vi "按日期零件型号保存图片.vi"(8 "结果":bool, 9 "当前零件型号":string, 10 "选项":T2(ring), 11 "Img in":T1) -> ()   [LabVIEW 2014]
uses:
  Global.vi
  <vilib>/vision/Image Controls.llb/IMAQ Image.ctl
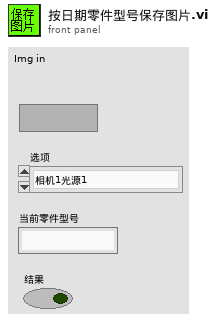
[diagram p1: front panel]
types:
  T1 = typedef "IMAQ Image.ctl" = refnum<image>
  T2 = enum16{"相机1光源1", "相机1光源2", "相机2光源3", "相机2光源4", "相机3光源5", "相机3光源6"}
  T3 = typedef "OtherSpec.ctl" = cluster{"其它勾选类规格":T4, "其它数据类规格":T5, "相机名称":T6}
  T4 = typedef "其它勾选类规格.ctl" = cluster{"保存NG图片":bool, "保存OK图片":bool, "保存数据":bool, "开机默认开启监控摄像头":bool}
  T5 = typedef "其他数据类规格.ctl" = cluster{"相机1像素-毫米换算系数":dbl, "相机2像素-毫米换算系数":dbl, "D盘剩余空间预警(G)":dbl, "视频最长录制时间(秒)":dbl}
  T6 = typedef "相机名称品牌使用状态.ctl" = cluster{"相机1名称":T7, "相机2名称":T7, "Cam1启用":bool, "Cam2启用":bool, "Basler1":bool, "Basler2":bool}
  T7 = typedef "IMAQdx.ctl" = refnum<k21>
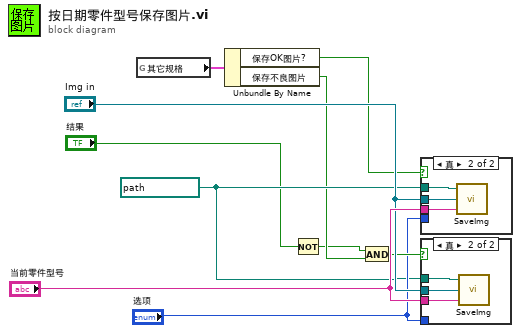
[diagram p0: block diagram]
diagram:
  w6 = path "D:/测试图片" ("Cam1Light1SavePath")
  n1 = global read "Global.vi" "其它规格"() -> (w5:T3)
  n2 = Unbundle By Name(w5) -> ("保存OK图片?"=w4:bool, "保存不良图片"=w3:bool)
  n3 = Not(x="结果") -> (.not. x?=w1:bool)
  n4 = And(x=w1, y=w3) -> (x .and. y?=w8:bool)
  n5 = case shown="真" w4 {
    tunnel: w6 -> [_ w13]
    tunnel: "当前零件型号" -> [_ w12]
    tunnel: "Img in" -> [_ w11]
    tunnel: "选项" -> [_ _]
    frame False {
    }
    frame True {
      n6 = call "SaveImg.vi"("零件型号"=w12, "Image"=w11, "Fold路径"=w13) -> ()
    }
  }
  n7 = case shown="真" w8 {
    tunnel: w6 -> [_ w16]
    tunnel: "当前零件型号" -> [_ w15]
    tunnel: "Img in" -> [_ w14]
    tunnel: "选项" -> [_ _]
    frame False {
    }
    frame True {
      n8 = call "SaveImg.vi"("零件型号"=w15, "Image"=w14, "Fold路径"=w16) -> ()
    }
  }
